vi "test Write and Read Signed Integer.vi"(8 "error in (no error)":errorcluster, 11 "TestCase in":refnum<class "Read Value Tests.lvclass">) -> (0 "error out":errorcluster, 3 "TestCase out":refnum<class "Read Value Tests.lvclass">)   [LabVIEW 2017, in "Mem Buff Tests.lvlib" / "Read Value Tests.lvclass"]
uses:
  Read Value Tests.lvclass
  Read Value Tests.lvclass/Read Value Tests.ctl
  Engine/Classes/Buffer/Read 0D I8.vi
  Engine/Classes/Buffer/Read 0D I16.vi
  Engine/Classes/Buffer/Read 0D I32.vi
  Engine/Classes/Buffer/Read 0D I64.vi
  <vilib>/addons/_JKI Toolkits/VI Tester/TestCase.llb/TestCase.lvclass
  Engine/Classes/Buffer/Buffer.lvclass
  C:/Program Files (x86)/National Instruments/LabVIEW 2017/vi.lib/addons/_JKI Toolkits/VI Tester/TestCase.llb/TestCase.lvclass
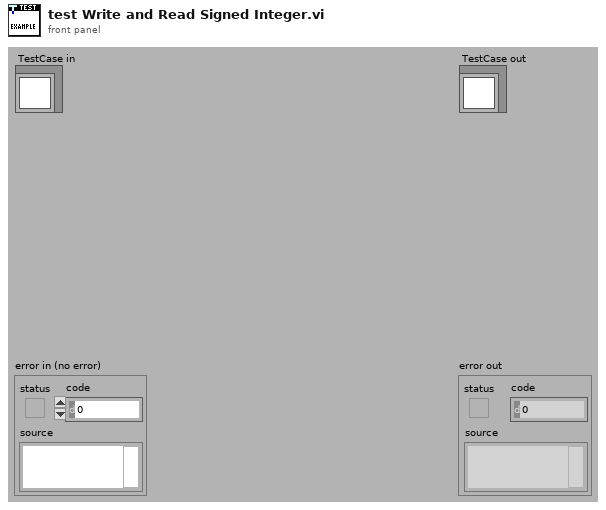
[diagram p1: front panel]
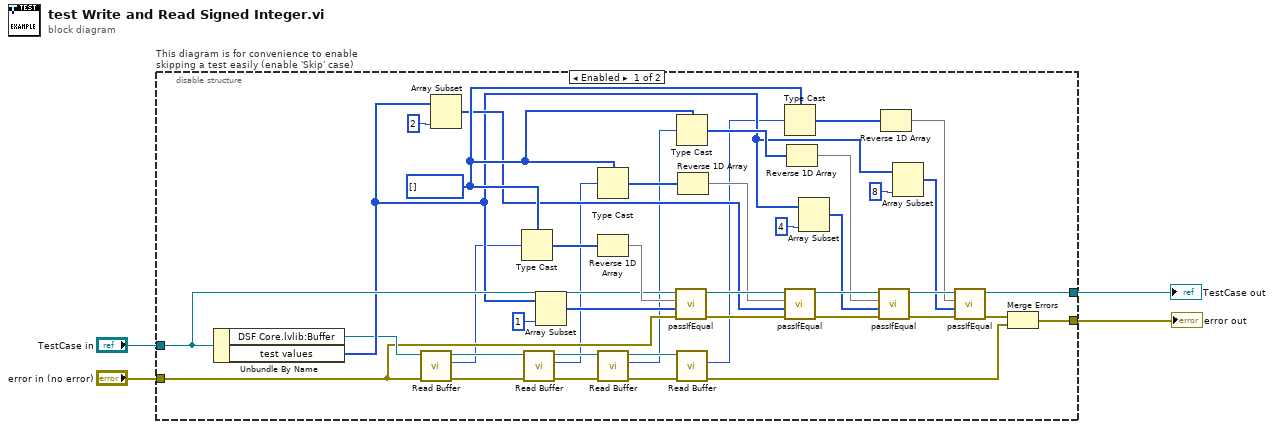
[diagram p0: block diagram]
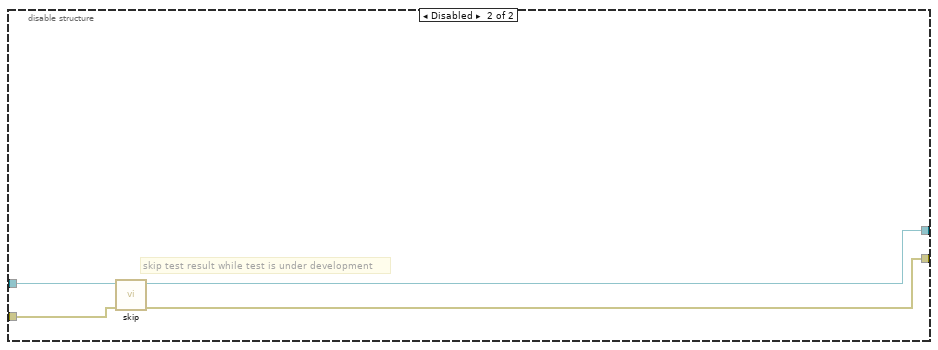
[diagram p2: hidden frame]
diagram:
  n1 = disable-structure "This diagram is for convenience to enable skipping a test easily (enable 'Skip' case)" shown="Enabled" {
    disable-tunnel: "TestCase in" -> [w14 w49]
    disable-tunnel: [w15 w47] -> w2
    disable-tunnel: [w10 w48] -> w3
    disable-tunnel: "error in (no error)" -> [w11 w46]
    frame Enabled {
      w32 = u8[] [] ("buffer in")
      n2 = Unbundle By Name(w14) -> ("DSF Core.lvlib:Buffer"=w12:refnum<class "Buffer.lvclass">, "test values"=w13:u8[])
      n3 = call-poly "Read Buffer.vi"("error in (no error)"=w11, "Buffer in"=w12) -> ("error out"=w41:errorcluster, "value out"=w8:i8, "Buffer out"=w42:refnum<class "Buffer.lvclass">)  [unwired: 6 in, 1 out]
      n4 = Array Subset(array=w13, length=2) -> (w21:u8[])  [unwired: 1 in]
      n5 = Type Cast(type=w32, x=w8) -> (*(type *) &x=w36:u8[])
      n6 = call-poly "Read Buffer.vi"("error in (no error)"=w41, "Buffer in"=w42) -> ("error out"=w39:errorcluster, "value out"=w7:i16, "Buffer out"=w40:refnum<class "Buffer.lvclass">)  [unwired: 6 in, 1 out]
      n7 = Array Subset(array=w13, length=1) -> (w22:u8[])  [unwired: 1 in]
      n8 = Type Cast(type=w32, x=w7) -> (*(type *) &x=w35:u8[])
      n9 = Reverse 1D Array(array=w36) -> (reversed array=w24:u8[])
      n10 = call-poly "Read Buffer.vi"("error in (no error)"=w39, "Buffer in"=w40) -> ("error out"=w37:errorcluster, "value out"=w6:i32, "Buffer out"=w38:refnum<class "Buffer.lvclass">)  [unwired: 6 in, 1 out]
      n11 = call-dynamic "passIfEqual.vi"("error in (no error)"=w11, "y"=w22, "x"=w24, "TestCase in"=w14) -> ("error out"=w27:errorcluster, "TestCase out"=w28:refnum<class "Read Value Tests.lvclass">)  [unwired: 6 in]
      n12 = Type Cast(type=w32, x=w6) -> (*(type *) &x=w34:u8[])
      n13 = call-poly "Read Buffer.vi"("error in (no error)"=w37, "Buffer in"=w38) -> ("error out"=w9:errorcluster, "value out"=w5:i64)  [unwired: 6 in, 2 out]
      n14 = Reverse 1D Array(array=w35) -> (reversed array=w23:u8[])
      n15 = Type Cast(type=w32, x=w5) -> (*(type *) &x=w33:u8[])
      n16 = call-dynamic "passIfEqual.vi"("error in (no error)"=w27, "y"=w21, "x"=w23, "TestCase in"=w28) -> ("error out"=w25:errorcluster, "TestCase out"=w26:refnum<class "Read Value Tests.lvclass">)  [unwired: 6 in]
      n17 = Reverse 1D Array(array=w34) -> (reversed array=w19:u8[])
      n18 = Array Subset(array=w13, length=4) -> (w20:u8[])  [unwired: 1 in]
      n19 = call-dynamic "passIfEqual.vi"("error in (no error)"=w25, "y"=w20, "x"=w19, "TestCase in"=w26) -> ("error out"=w30:errorcluster, "TestCase out"=w29:refnum<class "Read Value Tests.lvclass">)  [unwired: 6 in]
      n20 = Reverse 1D Array(array=w33) -> (reversed array=w17:u8[])
      n21 = Array Subset(array=w13, length=8) -> (w18:u8[])  [unwired: 1 in]
      n22 = call-dynamic "passIfEqual.vi"("error in (no error)"=w30, "y"=w18, "x"=w17, "TestCase in"=w29) -> ("error out"=w16:errorcluster, "TestCase out"=w15:refnum<class "Read Value Tests.lvclass">)  [unwired: 6 in]
      n23 = Merge Errors(w16, w9) -> (w10:errorcluster)
    }
    frame Disabled {
      # "skip test result while test is under development"
      n24 = call <vilib>:"skip.vi"("error in (no error)"=w46, "TestCase in"=w49) -> ("error out"=w48:errorcluster, "TestCase out"=w47:refnum<class "Read Value Tests.lvclass">)  [unwired: 8 in]
    }
  }
  "error out" <- w3
  "TestCase out" <- w2
